vi "DMM multi test with switch.vi"() -> ()   [LabVIEW 2019]
uses:
  Chart_Graph_Mean_Range_StdDev.ctl
  <vilib>/Analysis/baseanly.llb/Mean (DBL).vi
  <vilib>/Analysis/NI_AALBase.lvlib
panel:
  in  "DMM 7.5 Digits All 4 Channels":dbl[][](array[numeric])=[[3.4835981189908805, 3.4835973578772146, 3.4835977893402292, 3.483597533766503, 3.4835975009361055, 3.4835974259988975, 3.4835978392404665, 3.483597710153336, 3.483597530409142, 3.483597982965577, 3.4835974835927273, 3.4835975661067864, 3.4835978929675346, 3.483597859704548, 3.483597570043803, 3.48359758877419, 3.483597718635417, 3.4835974386993853, 3.4835979909144443, 3.483597546796911, 3.483597791629489, 3.4835976928422, 3.4835977006392365, 3.4835976984527726, 3.4835973562416775, 3.483597995505588, 3.483597815535534, 3.4835978300326116, 3.483597985892642, 3.483597413809255, 3.483597723962119, 3.4835979022635915, 3.4835977166666647, 3.483597588468151, 3.483598009044623, 3.4835974566412133, 3.4835975839370192, 3.4835975376641026, 3.483597439503911, 3.483597317956866, 3.4835972485909776, 3.4835976458862903, 3.4835976825108617, 3.48359823081158, 3.4835976718930137, 3.4835976585808193, 3.4835978362135966, 3.483597507818025, 3.483597799164003, 3.483597349716458, 3.4835975948182454, 3.4835981329699433, 3.4835979467910407, 3.4835974912342884, 3.4835974532960456, 3.483597903200004, 3.483597374049583, 3.483597334623242, 3.483597710860957, 3.483597692009984, 3.4835976586327315, 3.4835977598936534, 3.4835979763023603, 3.4835975896116587, 3.4835978971434263, 3.4835976281822316, 3.4835982271082013, 3.4835976949272403, 3.4835974320575938, 3.483597408013519, 3.4835976534048685, 3.48359766337321, 3.483597430968089, 3.4835978228589006, 3.4835977691488273, 3.4835979109499484, 3.483597518460395, 3.483597806961959, 3.483597578691926, 3.4835975527599476, 3.483597860450459, 3.4835974511972227, 3.4835973978219275, 3.4835975280386107, 3.4835970961662297, 3.4835979186960975, 3.483597285920934, 3.483597386907896, 3.483597474535041, 3.4835973080741587, 3.4835975196582534, 3.4835974480673357, 3.4835976798422204, 3.483597547235268, 3.483597484346667, 3.483597539878841, 3.483597791092996, 3.483597598658644, 3.48359767066429, 3.4835976010356733, 3.4835977898228307, 3.483597544054286, 3.4835971331899516, 3.4835975044953993, 3.4835974626533996, 3.483597132727585, 3.4835975524889027, 3.4835979535117207, 3.4835972493429948, 3.483597640255253, 3.4835974086907697, 3.4835973506672318, 3.483597580088908, 3.483597239500539, 3.483597486011177, 3.4835975002194246, 3.483597090891085, 3.483597714859873, 3.4835976666442754, 3.4835972680152745, 3.4835977448807194, 3.483597350763673, 3.4835973529914943, 3.4835976118884404, 3.4835975154265597, 3.483597695000821, 3.4835974558961684, 3.483597790103636], [3.4850700897521563, 3.485070233425622, 3.4850703496943347, 3.4850708481529473, 3.485070572181595, 3.485070105960937, 3.485070465485683, 3.4850704480083396, 3.48507056459965, 3.4850708183835595, 3.4850708166846527, 3.485070796405387, 3.4850707761851427, 3.485070608667662, 3.4850707882696508, 3.4850707241151975, 3.4850706596362566, 3.48507073021978, 3.485070567481813, 3.4850707162760663, 3.485070893790592, 3.4850704393547267, 3.485070651192876, 3.485070267833332, 3.4850708914554103, 3.4850705970227684, 3.4850705496821712, 3.485070893808849, 3.485070908236491, 3.4850704723673553, 3.4850706194869305, 3.4850704541132527, 3.4850707021341325, 3.4850710097049173, 3.4850709609995607, 3.4850706992583946, 3.4850710502732944, 3.4850708242361663, 3.485071009568022, 3.4850706205187802, 3.4850704634402474, 3.4850708131553314, 3.485070283346761, 3.485070802639425, 3.4850707294320875, 3.4850710718142284, 3.48507067385808, 3.4850708139996227, 3.4850706485313316, 3.485071205234073, 3.4850708802082133, 3.485070539592214, 3.4850703284695643, 3.485070644610402, 3.4850706377352365, 3.485070724333666, 3.485070706865352, 3.485071039978291, 3.4850708932740937, 3.4850703374231804, 3.4850706519379795, 3.4850704993977777, 3.4850704497575355, 3.4850705472916865, 3.4850708830277983, 3.4850702392811503, 3.48507065435932, 3.4850707605356352, 3.4850706390730855, 3.4850704744759575, 3.4850708749760537, 3.4850704959682712, 3.48507057686368, 3.485070482100544, 3.485070110520969, 3.4850708314094643, 3.4850704513493116, 3.485070655338042, 3.4850698942787095, 3.485070641499467, 3.485070060001174, 3.485070454200556, 3.485070688596838, 3.4850706243046936, 3.485070579152903, 3.485069883099495, 3.485070062034084, 3.485070525913557, 3.485070210088132, 3.485070026034661, 3.4850702456185907, 3.485070243940185, 3.4850697001719446, 3.4850702521018917, 3.4850700772887624, 3.4850700859590287, 3.485070371774776, 3.4850700961734526, 3.485070172855618, 3.485069905757029, 3.4850703159307965, 3.4850698537426226, 3.485070462070553, 3.4850699512833727, 3.4850698464028094, 3.4850699259717026, 3.4850701371431896, 3.4850702401475635, 3.485070006300969, 3.485070088453557, 3.4850701595221656, 3.485070253223072, 3.4850696208469243, 3.4850698353777982, 3.48506973491397, 3.4850699043293396, 3.485069909154778, 3.485069945468628, 3.4850700162729797, 3.4850700637961176, 3.4850698568711835, 3.485069683841688, 3.485069930522382, 3.48506970179727, 3.485070116146578, 3.485070421850128, 3.485070158963441, 3.4850698427039397], [3.481571899555477, 3.4815720996809536, 3.481572168540679, 3.481572401004205, 3.4815723090577384, 3.481571988546094, 3.4815728274152624, 3.4815728062014335, 3.481572501577856, 3.481572607429995, 3.481572610595567, 3.4815725639158046, 3.4815731629523547, 3.48157245445838, 3.481572678822192, 3.481572529789867, 3.4815725819006804, 3.481572967069484, 3.4815731074475686, 3.481572693006066, 3.4815728208347263, 3.481572524099559, 3.481573131123811, 3.4815725324422293, 3.4815725721654815, 3.4815727955137086, 3.4815732409351097, 3.48157252834275, 3.481572511998337, 3.4815730302590793, 3.481572830362119, 3.4815731395241, 3.48157304282813, 3.481573010928663, 3.4815726753855367, 3.481573126747513, 3.4815728716190883, 3.481572781318836, 3.481572732683734, 3.4815727357820037, 3.481572704616765, 3.481572784355119, 3.4815728763523865, 3.4815728056849347, 3.481572474565925, 3.4815728651620326, 3.481572960730617, 3.4815730411537085, 3.4815726474348017, 3.4815728656925575, 3.4815728037625746, 3.4815725683714147, 3.4815727765135653, 3.481572602782018, 3.4815725196736356, 3.4815723014267093, 3.481572220656706, 3.481572534362172, 3.4815728413086053, 3.481572371815714, 3.481572564065832, 3.4815724851708483, 3.4815726220738314, 3.481572401586816, 3.481572213900522, 3.481572531080011, 3.4815726736061214, 3.481572174946321, 3.4815728025844557, 3.481572249370352, 3.4815721671205733, 3.481572565457693, 3.481572360373885, 3.4815726824797832, 3.481572841781139, 3.481572643049169, 3.4815721595516465, 3.4815723952810407, 3.481572162387346, 3.4815727239032985, 3.4815723917459103, 3.4815720794809555, 3.4815722693538627, 3.4815725743888026, 3.4815720485747352, 3.481572470689445, 3.4815725915569478, 3.4815727324723182, 3.4815724521032285, 3.4815727954319797, 3.4815721995573847, 3.4815721839029323, 3.4815721980816043, 3.4815721160737434, 3.481572277861212, 3.4815721507038226, 3.481572288856155, 3.481572226063303, 3.4815719656002706, 3.481572592875911, 3.481572194406493, 3.481572412416302, 3.481572084967407, 3.4815721696802724, 3.4815720226137596, 3.48157205650772, 3.48157190538414, 3.481572045063342, 3.481572018317761, 3.481572185489624, 3.481572154901699, 3.481571926660422, 3.4815718999626237, 3.4815721280737373, 3.481572224094029, 3.481572353081591, 3.481572261017972, 3.481571975995548, 3.481572128201471, 3.481572180067718, 3.4815715655143373, 3.4815718214629943, 3.4815715789142585, 3.4815719255662994, 3.4815718246399183, 3.481571977351035, 3.481571843104722, 3.4815719523213], [3.484305724115568, 3.4843058305875227, 3.4843062901111512, 3.484305936231965, 3.4843057288438772, 3.4843064559020687, 3.4843063293991383, 3.4843062952127486, 3.4843066955825175, 3.484306829330163, 3.4843061981418333, 3.4843063620415697, 3.484306236532934, 3.4843064437456763, 3.4843061743985606, 3.484306186782022, 3.484306270580653, 3.484306740665737, 3.4843061208250283, 3.484305965882024, 3.484306590076414, 3.4843059649148156, 3.4843062673844587, 3.4843060655731373, 3.484306302924423, 3.484306432337808, 3.484306632080742, 3.484306009373001, 3.484306543172826, 3.484306382441485, 3.4843062427876945, 3.4843061764316796, 3.48430660308128, 3.4843062004511594, 3.4843060610943404, 3.4843068333436076, 3.484306621812408, 3.484306649840404, 3.484306285295565, 3.4843059813072683, 3.484306553789793, 3.4843062824735846, 3.484306430756184, 3.4843068757434295, 3.484306442887929, 3.4843065762633945, 3.484305988738697, 3.4843066243270724, 3.484306445500346, 3.484306832441937, 3.4843060150056067, 3.4843063781220796, 3.4843066789757673, 3.4843064150739504, 3.4843061381565823, 3.484305675942912, 3.4843062793645334, 3.4843063841371547, 3.484306272484438, 3.4843062706304226, 3.484306376440192, 3.484305708893772, 3.484306251000281, 3.484306233665289, 3.4843063068999873, 3.4843062524955, 3.4843063590903363, 3.484305999586689, 3.4843062500567994, 3.4843060777149777, 3.484305966811333, 3.4843060316739654, 3.4843057546627394, 3.484306023228924, 3.4843061239924005, 3.4843060196427316, 3.4843055330739823, 3.4843056881987136, 3.484305713110319, 3.484306038013802, 3.484305910294656, 3.4843055487391927, 3.484305955637334, 3.4843058755725593, 3.4843058736827315, 3.4843058395981483, 3.4843057942888587, 3.4843056863141157, 3.484305964223715, 3.4843061658501737, 3.4843061897594634, 3.484305738279498, 3.484305518799016, 3.484305825857164, 3.484306035291972, 3.484306102538148, 3.484305819322618, 3.4843057482448683, 3.4843055381532038, 3.484305561533999, 3.48430561697876, 3.484305709331289, 3.484305709513193, 3.4843057764415675, 3.484305845716869, 3.4843058548617227, 3.4843058558332802, 3.4843060036480638, 3.484306017456, 3.4843051117756003, 3.4843054695551543, 3.484305914306639, 3.4843058242771217, 3.4843058614305953, 3.4843052097363807, 3.4843056026459474, 3.484305395133235, 3.4843055297155088, 3.484305541519446, 3.4843059349268186, 3.4843053694848685, 3.4843057348549347, 3.484305160045847, 3.484304944580094, 3.4843056614719075, 3.4843052011624254, 3.4843052966632158, 3.484305352531343]]
  in  "Take New DMM 7.5 Digit Measurements":bool
  out "error values of channels":dbl[][](array[numeric])=[[3.088515718241425e-05, 2.4263952214553797e-05, 4.612398782866123e-05, 1.535158323395791e-05], [3.1800201541809514e-05, 2.555652910452011e-05, 4.833513349788987e-05, 1.7629648504602358e-05], [3.2785703003135325e-05, 2.681542600679876e-05, 5.033514020125196e-05, 1.9721279010731507e-05], [3.2754188132866346e-05, 2.6800178063446367e-05, 5.076858738028989e-05, 2.0244840135408282e-05], [3.2835440087364276e-05, 2.6995210473224063e-05, 5.1309970349411316e-05, 2.090291011525025e-05], [3.705956659905141e-05, 3.1461577734148705e-05, 5.597125976164463e-05, 2.561413463020301e-05], [3.403626202214127e-05, 2.8308646536245874e-05, 5.290407193214719e-05, 2.2366019222896938e-05], [2.454027838316719e-05, 1.8945226556432715e-05, 4.372569679533811e-05, 1.3596613212651931e-05], [3.582435173266063e-05, 3.0741277314394466e-05, 5.5675506236863015e-05, 2.4769572306126975e-05], [3.496152187887347e-05, 2.9052046070177084e-05, 5.39118719058429e-05, 2.4362891539286835e-05], [2.9893162372562898e-05, 2.429213407761921e-05, 4.9712756616582254e-05, 1.7854232706948636e-05], [3.364391183557913e-05, 2.464309119609709e-05, 4.3097751809551e-05, 1.2435587404713289e-05]] format="%#_6p"
  out "DMM mean values of channels":dbl[][](array[numeric])=[[3.4835667290651937, 3.4850461695956385, 3.4815263291466074, 3.484290688473681], [3.4835658140208343, 3.4850448770187485, 3.481524118000938, 3.48428841040841], [3.483564828519373, 3.4850436181218463, 3.481522117994235, 3.484286318777904], [3.4835648600342433, 3.4850436333697896, 3.481521684547056, 3.4842857952167794], [3.4835647787822888, 3.48504343833738, 3.4815211431640867, 3.4842851371467995], [3.483560554655777, 3.485038971970119, 3.4815164818746744, 3.4842804259222846], [3.483563577960354, 3.485042124901317, 3.481519549062504, 3.484283674037692], [3.483573073943993, 3.4850514883212966, 3.4815287274376407, 3.484292443443702], [3.4835617898706435, 3.4850396922705387, 3.481516777628199, 3.4842812704846087], [3.4835626527004973, 3.485041381501783, 3.4815185412625302, 3.4842816771653755], [3.4835677210600036, 3.4850461414137754, 3.4815227403778195, 3.484288185824208], [3.4835639703105405, 3.485045790456657, 3.4815293553826265, 3.48429360446951]] format="%#_6p"
  out "Results Output":T1={"ch3 range"=2.7418730868866703e-05, "ch3 std dev"=8.019227381292095e-06, "ch3 mean"=3.48429360446951, "Histogram Graph ch3"={"X Values"=[3.4842822002093103, 3.484284942082397, 3.4842876839554844, 3.484290425828571, 3.484293167701658, 3.4842959095747448, 3.4842986514478316, 3.484301393320919, 3.4843041351940056, 3.4843068770670924], "Histogram: h(x)"=[4, 5, 1, 3, 4, 3, 3, 4, 3, 2]}, "ch2 range"=3.540735570162212e-05, "ch2 std dev"=9.099200658741097e-06, "ch2 mean"=3.4815293553826265, "Histogram Graph ch2"={"X Values"=[3.4815133882246614, 3.4815169289602315, 3.4815204696958015, 3.4815240104313716, 3.4815275511669417, 3.481531091902512, 3.4815346326380823, 3.4815381733736523, 3.4815417141092224, 3.4815452548447925], "Histogram: h(x)"=[3, 1, 1, 6, 5, 6, 4, 1, 2, 3]}, "ch1 range"=2.735773523188101e-05, "ch1 std dev"=6.5501310918820285e-06, "ch1 mean"=3.485045790456657, "Histogram Graph ch1"={"X Values"=[3.4850333381714784, 3.4850360739450017, 3.4850388097185245, 3.485041545492048, 3.485044281265571, 3.4850470170390944, 3.4850497528126176, 3.4850524885861405, 3.4850552243596638, 3.485057960133187], "Histogram: h(x)"=[1, 1, 4, 5, 5, 7, 3, 1, 3, 2]}, "ch0 range"=4.1823320245271134e-05, "ch0 std dev"=1.0492211728305467e-05, "ch0 mean"=3.4835639703105405, "Histogram Graph ch0"={"X Values"=[3.483546101718765, 3.4835502840507893, 3.483554466382814, 3.4835586487148387, 3.483562831046863, 3.4835670133788876, 3.483571195710912, 3.4835753780429366, 3.4835795603749613, 3.4835837427069856], "Histogram: h(x)"=[1, 4, 5, 4, 2, 4, 6, 3, 2, 1]}, "Waveform Chart ch1"=[3.4850480524060563, 3.485045722429083, 3.485037882081368, 3.4850591458358426, 3.4850471789599404, 3.4850472572160394, 3.485045074452979, 3.4850404751072204, 3.4850461000410506, 3.485031970284717, 3.485045322781052, 3.485038507352649, 3.485055795569339, 3.485041625145203, 3.485055278526134, 3.485041729761377, 3.4850380638078504, 3.485046785956284, 3.485050493636467, 3.4850434541169735, 3.4850503736265135, 3.4850476055501556, 3.4850593280199487, 3.485042782830599, 3.4850409420954906, 3.4850386197204175, 3.485045389162435, 3.4850541443324676, 3.4850347239163444, 3.485050168037523, 3.4850439475642583, 3.4850513542892396], "Waveform Chart ch2"=[3.481515607361682, 3.481527404166462, 3.4815303118947307, 3.4815470252125778, 3.4815274259590856, 3.4815255492194326, 3.4815302697552184, 3.48152318249469, 3.4815260878164613, 3.4815251999463683, 3.481526915907382, 3.481535193911727, 3.4815309448763383, 3.481529469056688, 3.481545439354732, 3.481511617856876, 3.481540697335584, 3.481524235529164, 3.481542476984634, 3.481526181645006, 3.481535707797748, 3.4815150651586197, 3.4815222983196796, 3.481535652607903, 3.481521749482858, 3.4815310736450336, 3.48153627048455, 3.4815442684817395, 3.4815237249905873, 3.4815308967097223, 3.481511934166034, 3.4815394941147297], "Waveform Chart ch0"=[3.483585833872998, 3.4835617549981377, 3.4835593509805425, 3.483555132097129, 3.483575280342153, 3.4835645353108147, 3.4835799618069827, 3.4835440105527526, 3.4835724068287552, 3.483557714524022, 3.4835716013232054, 3.4835554574069376, 3.483568514630331, 3.4835499192040302, 3.4835683163469238, 3.4835712287954164, 3.4835693926823277, 3.483558447252551, 3.4835584584629746, 3.4835672300687337, 3.4835503673913766, 3.4835705222977005, 3.483556539604654, 3.4835813453087714, 3.483549944163877, 3.4835666357823585, 3.4835524119001446, 3.4835761177139886, 3.4835546044996337, 3.483575038372925, 3.4835493393306862, 3.4835696360834634], "Waveform Chart ch3"=[3.484284886270981, 3.484302769126643, 3.484292687483238, 3.48430577464466, 3.4842826507236904, 3.484298595774609, 3.4842817990987145, 3.484304482713164, 3.4842878879424797, 3.4842948090081647, 3.4842838250157917, 3.484301294571594, 3.4842990834396947, 3.4842926245411245, 3.4843008439293763, 3.484292166755767, 3.484308248003636, 3.484284987307844, 3.484300544819285, 3.484280829272767, 3.4843022842457367, 3.484291127833416, 3.484304774105647, 3.4842858995893384, 3.48429959601284, 3.4842915595411452, 3.4842950842058777, 3.48429585576079, 3.4842847505352093, 3.4842891151931603, 3.484280939709867, 3.484293565848077]} {"ch3 range" format="%#_6p"; "ch3 std dev" format="%#.3p"; "ch3 mean" format="%#.6p"; "ch2 range" format="%#_6p"; "ch2 std dev" format="%#.3p"; "ch2 mean" format="%#.6p"; "ch1 range" format="%#_6p"; "ch1 std dev" format="%#.3p"; "ch1 mean" format="%#.6p"; "ch0 range" format="%#_6p"; "ch0 std dev" format="%#.3p"; "ch0 mean" format="%#.6p"}
  out "DMM Standard Deviation vs Aperture Time":T2(graph)={"Standard Deviation (Ohm)"=[0.0001, 0.0002, 0.001, 0.002, 0.005, 0.01, 0.016666666666666666, 0.03333333333333333, 0.05, 0.06666666666666667, 0.08333333333333333, 0.1], "Aperture Time (s)"=[8.521171410093747e-06, 8.355776903770358e-06, 5.957648703941697e-06, 5.648428795679757e-06, 5.083125453475177e-06, 4.220751270929592e-06, 2.5734818145425224e-06, 4.679098801087691e-07, 4.019467897813027e-07, 4.2762972154190507e-07, 3.674152693395681e-07, 4.1842664461027853e-07]}
  out "Aperture Time (s)":dbl[](array[numeric])=[0.0001, 0.0002, 0.001, 0.002, 0.005, 0.01, 0.016666666666666666, 0.03333333333333333, 0.05, 0.06666666666666667, 0.08333333333333333, 0.1] format="%#_6p"
  out "Sample Rates (Hz)":dbl[](array[numeric])=[10000.0, 5000.0, 1000.0, 500.0, 200.0, 100.0, 60.0, 30.0, 20.0, 15.0, 12.0, 10.0] format="%#_6p"
  out "Std Dev (V)":dbl[](array[numeric])=[8.521171410093747e-06, 8.355776903770358e-06, 5.957648703941697e-06, 5.648428795679757e-06, 5.083125453475177e-06, 4.220751270929592e-06, 2.5734818145425224e-06, 4.679098801087691e-07, 4.019467897813027e-07, 4.2762972154190507e-07, 3.674152693395681e-07, 4.1842664461027853e-07] format="%#_6p"
  out "Range (V)":dbl[](array[numeric])=[3.459052773857607e-05, 3.0322450345066088e-05, 2.0886762187366514e-05, 1.887653696641678e-05, 1.7470039061384668e-05, 1.3165505951651113e-05, 8.491743382466055e-06, 1.9452442872047726e-06, 1.6926320023369357e-06, 1.7219827928016684e-06, 1.5213698170146728e-06, 1.7526410622803468e-06] format="%#_6p"
  out "Elapsed Time (ms)":u32[](array[numeric])=[284, 309, 338, 482, 856, 1528, 2385, 4540, 6673, 8832, 10965, 13149]
  out "error out":errorcluster
  in  "error in":errorcluster
  in  "Rates":dbl[](array[numeric])=[10.0, 12.0, 15.0, 20.0, 30.0, 60.0, 100.0, 200.0, 500.0, 1000.0, 5000.0, 10000.0] format="%#_6p"
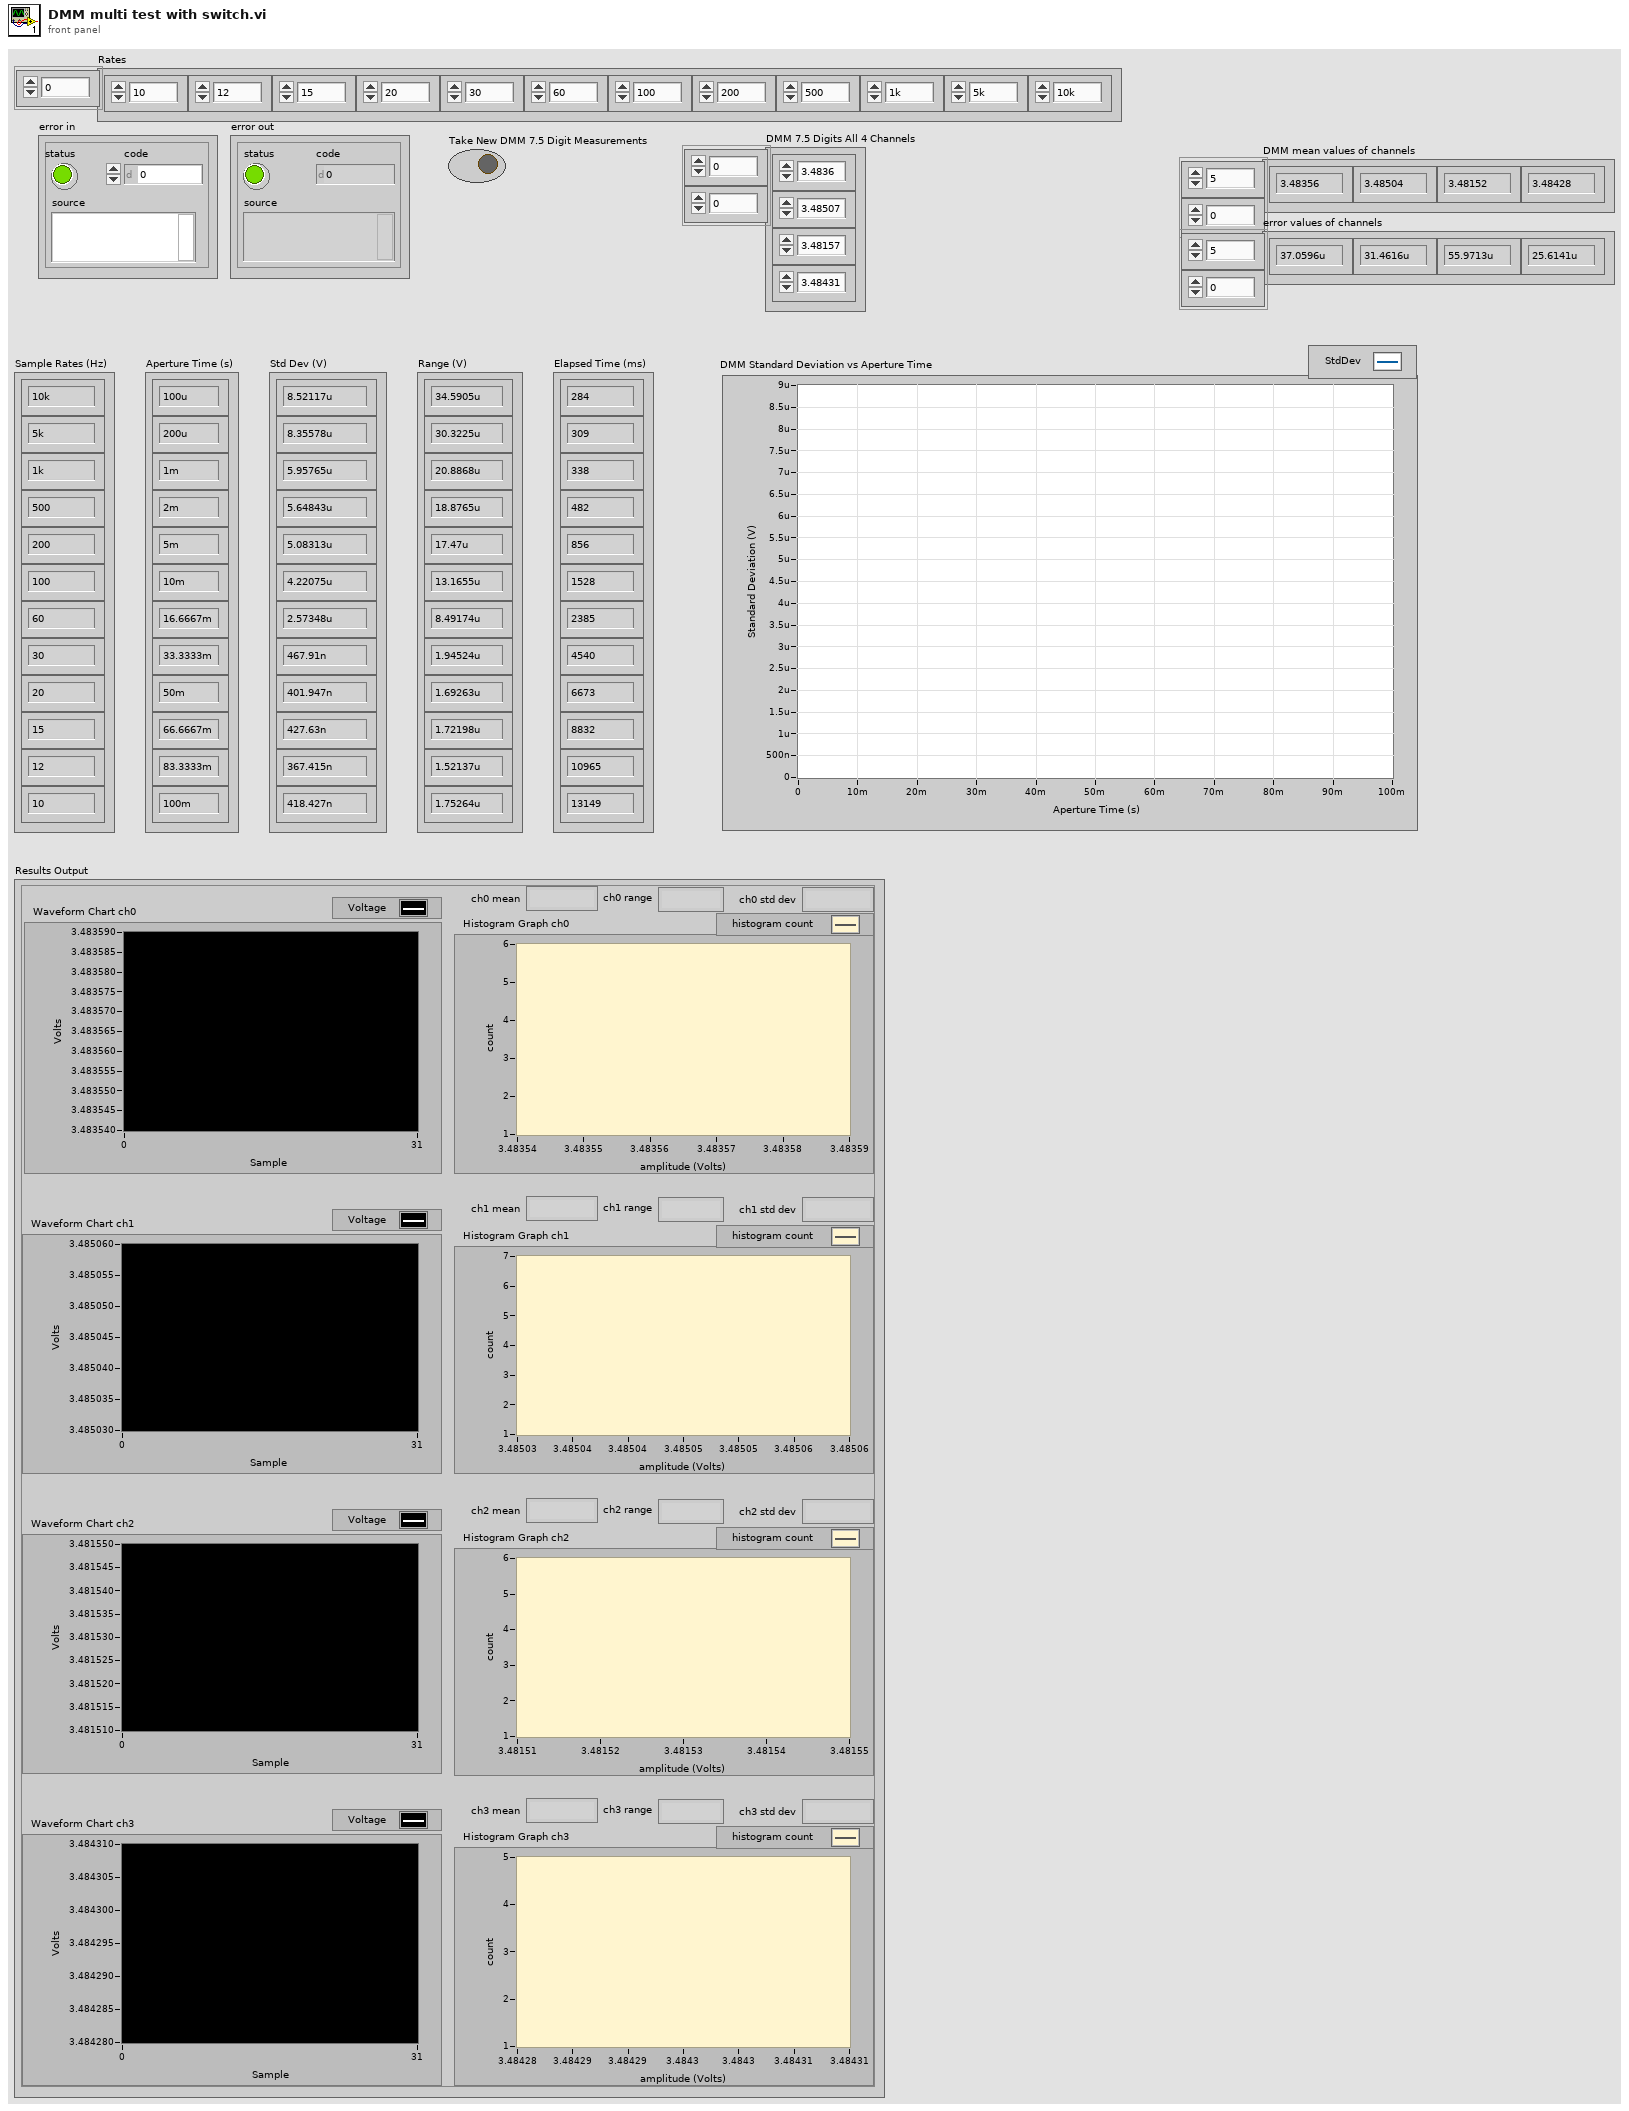
[diagram p1: front panel]
types:
  T1 = typedef "Chart_Graph_Mean_Range_StdDev.ctl" = cluster{"ch3 range":dbl, "ch3 std dev":dbl, "ch3 mean":dbl, "Histogram Graph ch3":cluster{"X Values":dbl[], "Histogram: h(x)":i32[]}, "ch2 range":dbl, "ch2 std dev":dbl, "ch2 mean":dbl, "Histogram Graph ch2":cluster{"X Values":dbl[], "Histogram: h(x)":i32[]}, "ch1 range":dbl, "ch1 std dev":dbl, "ch1 mean":dbl, "Histogram Graph ch1":cluster{"X Values":dbl[], "Histogram: h(x)":i32[]}, "ch0 range":dbl, "ch0 std dev":dbl, "ch0 mean":dbl, "Histogram Graph ch0":cluster{"X Values":dbl[], "Histogram: h(x)":i32[]}, "Waveform Chart ch1":dbl[], "Waveform Chart ch2":dbl[], "Waveform Chart ch0":dbl[], "Waveform Chart ch3":dbl[]}
  T2 = cluster{"Standard Deviation (Ohm)":dbl[], "Aperture Time (s)":dbl[]}
  T3 = typedef "OCVResults.ctl" = cluster{"V ch0 Array":dbl[], "V ch1 Array":dbl[], "V ch2 Array":dbl[], "V ch3 Array":dbl[], "V ch4 Array":dbl[], "Elapsed Time (ms)":u32, "DMM Fault Array":bool[]}
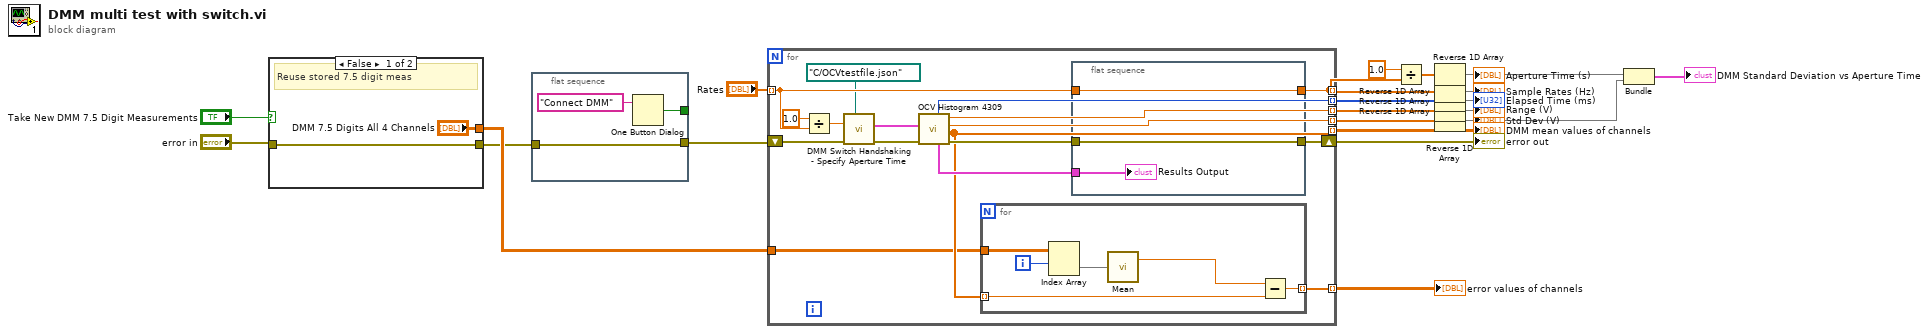
[diagram p0: block diagram]
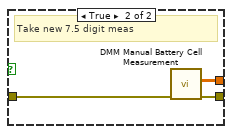
[diagram p2: hidden frame]
diagram:
  n1 = case shown="False" "Take New DMM 7.5 Digit Measurements" {
    tunnel: "error in" -> [w23 w26]
    tunnel: ["DMM 7.5 Digits All 4 Channels" w25] -> w11
    tunnel: [w23 w24] -> w10
    frame False {
      # "Reuse stored 7.5 digit meas"
    }
    frame True {
      # "Take new 7.5 digit meas"
      n2 = call "DMM Manual Battery Cell Measurement.vi"("error in"=w26) -> ("error out"=w24:errorcluster, "Measurements (Volts) All"=w25:dbl[][])  [unwired: 9 in]
    }
  }
  n3 = flat-sequence {
    tunnel: w10 -> [w28]
    tunnel: [w28] -> w9
    tunnel: [w27] -> _
    frame #0 {
      n4 = One Button Dialog(message="Connect DMM") -> (true=w27:bool)  [unwired: 1 in]
    }
  }
  n5 = for {
    shift-right: [w41] -> w21
    shift-left: w9 -> [w33]
    tunnel: [w46] -> w17 mode=indexing
    tunnel: [w45] -> w16 mode=indexing
    tunnel: [w44] -> w13 mode=indexing
    tunnel: [w39] -> w20 mode=indexing
    tunnel: [w40] -> w18 mode=indexing
    tunnel: "Rates" -> [w36] mode=indexing
    tunnel: [w38] -> w12 mode=indexing
    tunnel: w11 -> [w37]
    n6 = Divide(x=1.0, y=w36) -> (x/y=w31:dbl)
    n7 = call "DMM Switch Handshaking - Specify Aperture Time.vi"("error in"=w33, "Configuration:Advanced:Aperture Time"=w31, "file path (use dialog)"=path "C:/OCVtestfile.json") -> ("error out"=w34:errorcluster, "Results"=w32:T3)  [unwired: 7 in]
    n8 = call "OCV Histogram 4309.vi"("Error In"=w34, "Results Input"=w32) -> ("Error Out"=w42:errorcluster, "mean values of channels"=w39:dbl[], "std dev"=w44:dbl, "range"=w45:dbl, "Results Output"=w43:T1, "Elapsed Time (ms)"=w46:u32)  [unwired: 4 in]
    n9 = for {
      tunnel: w39 -> [w52] mode=indexing
      tunnel: [w51] -> w38 mode=indexing
      tunnel: w37 -> [w50]
      i -> [w49]
      n10 = Index Array(array=w50, index (row)=w49) -> (element=w48:dbl[])  [unwired: 1 in]
      n11 = call-poly <vilib>:"Mean.vi"("X"=w48) -> ("mean"=w47:dbl)  [unwired: 1 out]
      n12 = Subtract(x=w47, y=w52) -> (x-y=w51:dbl)
    }
    n13 = flat-sequence {
      tunnel: w43 -> [w55]
      tunnel: w42 -> [w54]
      tunnel: [w54] -> w41
      tunnel: w36 -> [w53]
      tunnel: [w53] -> w40
      frame #0 {
        "Results Output" <- w55
      }
    }
  }
  "error out" <- w21
  "DMM mean values of channels" <- w20
  "error values of channels" <- w12
  n14 = Divide(x=1.0, y=w18) -> (x/y=w14:dbl[])
  n15 = Reverse 1D Array(array=w14) -> (reversed array=w5:dbl[])
  "Aperture Time (s)" <- w5
  n16 = Reverse 1D Array(array=w18) -> (reversed array=→"Sample Rates (Hz)":dbl[])
  n17 = Reverse 1D Array(array=w17) -> (reversed array=→"Elapsed Time (ms)":u32[])
  n18 = Reverse 1D Array(array=w16) -> (reversed array=→"Range (V)":dbl[])
  n19 = Reverse 1D Array(array=w13) -> (reversed array=w1:dbl[])
  "Std Dev (V)" <- w1
  n20 = Bundle(w5, w1) -> (→"DMM Standard Deviation vs Aperture Time":cluster{dbl[], dbl[]})  [unwired: 1 in]
